vi "Dpc Get Dpc Version.vi"(8 "error in (no error)":errorcluster, 10 "perc":i32, 11 "szVersion":string) -> (0 "error out":errorcluster, 1 "function return":i32, 2 "perc out":i32, 3 "szVersion out":string)   [LabVIEW 2011, in "LVH-Adept.lvlib" / "DPCUTIL.lvlib"]
doc: "DPCAPI BOOL DpcGetDpcVersion(char * szVersion, ERC *perc);"
uses:
  DPCUTIL.lvlib
  dpcutil.dll
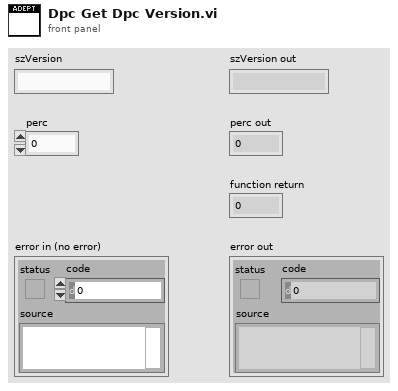
[diagram p1: front panel]
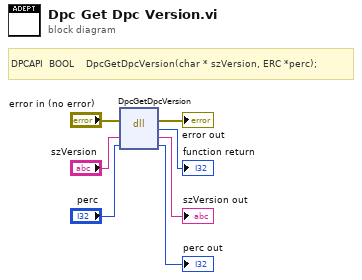
[diagram p0: block diagram]
diagram:
  # "DPCAPI  BOOL    DpcGetDpcVersion(char * szVersion, ERC *perc);"
  n1 = dll-call lib="dpcutil.*" fn="DpcGetDpcVersion"(error in="error in (no error)", "szVersion"="szVersion", "perc"="perc") -> (error out=→"error out":errorcluster, →"function return":i32, "szVersion"=→"szVersion out":string, "perc"=→"perc out":i32)  [unwired: 2 in, 1 out]
